vi "set_rois.vi"(0 "Tracker Handle":i32, 1 "Binning":i32, 2 "Array":dbl[][](array[numeric])) -> ()   [LabVIEW 2015]
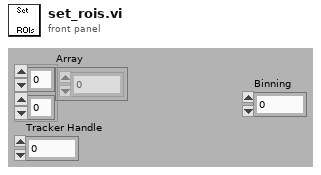
[diagram p1: front panel]
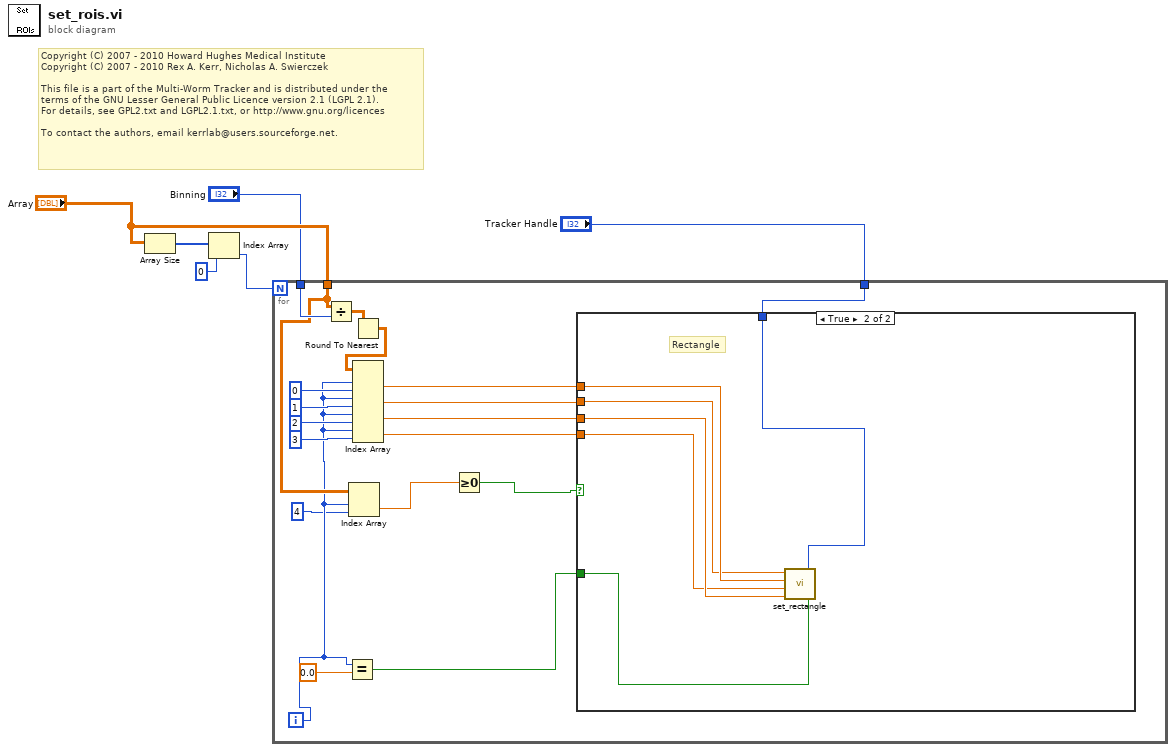
[diagram p0: block diagram]
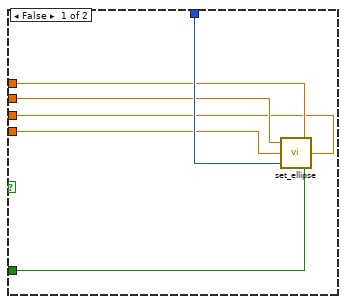
[diagram p2: hidden frame]
diagram:
  # "Copyright (C) 2007 - 2010 Howard Hughes Medical Institute\nCopyright (C) 2007 - 2010 Rex A. Kerr, Nicholas A. Swierczek\n \nThis file is a part of the Multi-Worm Tracker and is distributed under the\nterms of the GNU Lesser General Public Licence version 2.1 (LGPL 2.1).\nFor details, see GPL2.txt and LGPL2.1.txt, or http://www.gnu.org/licences\n \nTo contact the authors, email kerrlab@users.sourceforge.net."
  n1 = Array Size(array="Array") -> (size(s)=w5:i32[])
  n2 = Index Array(array=w5, index=0) -> (element=w6:i32)
  n3 = for {
    N: w6 -> [_]
    tunnel: "Array" -> [w10]
    tunnel: "Tracker Handle" -> [w23]
    tunnel: "Binning" -> [w13]
    i -> [w8]
    n4 = Divide(x=w10, y=w13) -> (x/y=w12:dbl[][])
    n5 = Equal?(x=w8, y=0.0) -> (x = y?=w24:bool)
    n6 = Index Array(array=w10, index (row)=w8, index (col)=4 ("disabled index (col)")) -> (element=w9:dbl)
    n7 = Round To Nearest(number=w12) -> (nearest integer value=w11:dbl[][])
    n8 = Index Array(array=w11, index (row) #1=w8, index (col) #1=0 ("disabled index (col)"), index (row) #2=w8, index (col) #2=1 ("disabled index (col)"), index (row) #3=w8, index (col) #3=2 ("disabled index (col)"), index (row) #4=w8, index (col) #4=3 ("disabled index (col)")) -> (element #1=w17:dbl, element #2=w16:dbl, element #3=w15:dbl, element #4=w14:dbl)
    n9 = Greater Or Equal To 0?(x=w9) -> (x >= 0?=w18:bool)
    n10 = case shown="True" w18 {
      tunnel: w24 -> [w31 w36]
      tunnel: w23 -> [w30 w37]
      tunnel: w17 -> [w29 w35]
      tunnel: w16 -> [w28 w34]
      tunnel: w15 -> [w27 w33]
      tunnel: w14 -> [w26 w32]
      frame False {
        n11 = call "set_ellipse.vi"("Set/Add"=w31, "y2"=w27, "y1"=w29, "Handle"=w30, "x2"=w26, "x1"=w28) -> ()
      }
      frame True {
        # "Rectangle"
        n12 = call "set_rectangle.vi"("Set/Add"=w36, "Handle"=w37, "y2"=w33, "x2"=w32, "y1"=w35, "x1"=w34) -> ()
      }
    }
  }
